vi "distance calculator.vi"(1 "Resolution Y":u16, 3 "Array":dbl[][](array[numeric])) -> (0 "Distances (Inches)":dbl)   [LabVIEW 2012]
doc: "Determines best target goal to calculate distance with, then uses bounding box top and bottom to calculate height. Determines distance by the formula:\ndistance = ( [ 1/2 ResolutionY * Goal size in inches] / Goal size in pixels ) / tan( 0.5 * Camera view angle)\nInputs: Goal Array (Portrait) & Image Resolution Y\nOutputs: Distance to Target (Inches)"
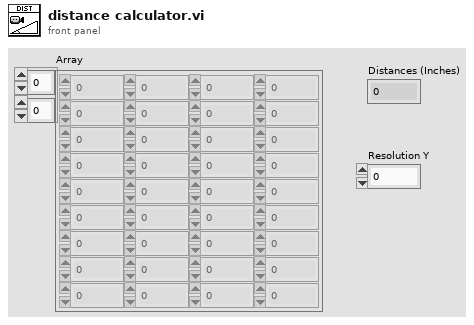
[diagram p1: front panel]
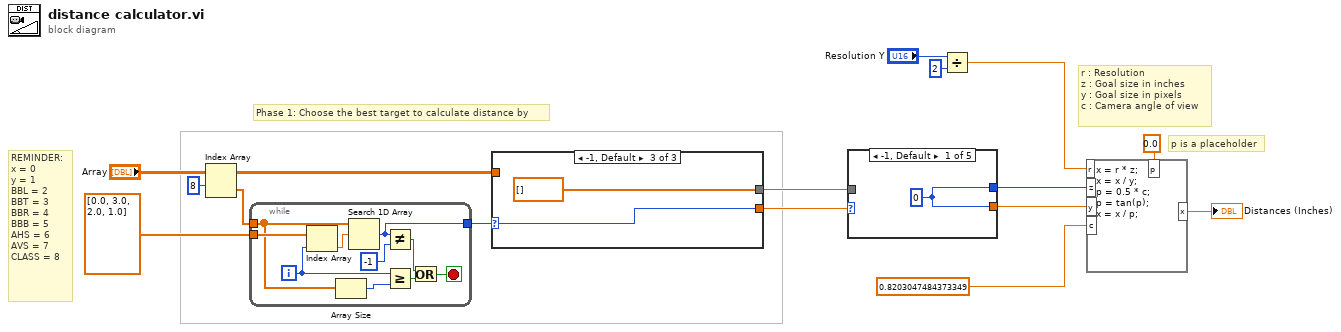
[diagram p0: block diagram]
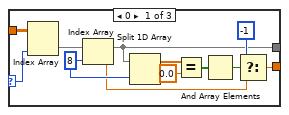
[diagram p2: hidden frame]
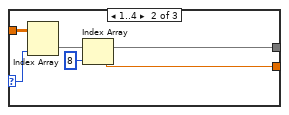
[diagram p3: hidden frame]
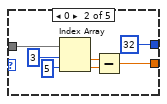
[diagram p4: hidden frame]
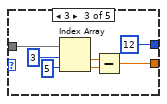
[diagram p5: hidden frame]
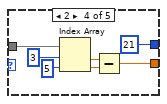
[diagram p6: hidden frame]
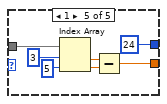
[diagram p7: hidden frame]
diagram:
  # "Phase 1: Choose the best target to calculate distance by"
  # "p is a placeholder"
  # "r : Resolution\nz : Goal size in inches\ny : Goal size in pixels\nc : Camera angle of view"
  # "REMINDER:\nx = 0\ny = 1\nBBL = 2\nBBT = 3\nBBR = 4 \nBBB = 5 \nAHS = 6\nAVS = 7 \nCLASS = 8"
  n1 = Index Array(array="Array", index (row)=8 ("disabled index (col)")) -> (element=w15:dbl[])  [unwired: 1 in]
  n2 = while {
    tunnel: w15 -> [w16]
    tunnel: dbl[] [0.0, 3.0, 2.0, 1.0] -> [w23]
    tunnel: [w24] -> w12
    i -> [w19]
    stop <- w21 stop-if-true
    n3 = Index Array(array=w23, index=w19) -> (element=w22:dbl)
    n4 = Array Size(array=w16) -> (size(s)=w18:i32)
    n5 = Search 1D Array(1D array=w16, element=w22) -> (index of element=w24:i32)  [unwired: 1 in]
    n6 = Not Equal?(x=w24, y=-1) -> (x != y?=w17:bool)
    n7 = Greater Or Equal?(x=w19, y=w18) -> (x >= y?=w20:bool)
    n8 = Or(x=w17, y=w20) -> (x .or. y?=w21:bool)
  }
  n9 = case shown="-1, Default" w12 {
    selector: w12 -> [w34 w39 w42]
    tunnel: "Array" -> [w35 w40 _]
    tunnel: [w28 w37 dbl[] [] ("Array")] -> w11
    tunnel: [w26 w38 w42] -> w5
    frame 0 {
      w33 = 8 ("index")
      n10 = Index Array(array=w35, index (col)=w34) -> (element=w28:dbl[])  [unwired: 1 in]
      n11 = Index Array(array=w28, index=w33) -> (element=w27:dbl)
      n12 = Split 1D Array(array=w28, index=w33) -> (first subarray=w32:dbl[])  [unwired: 1 out]
      n13 = Equal?(x=w32, y=0.0) -> (x = y?=w30:bool[])
      n14 = And Array Elements(Boolean array=w30) -> (logical AND=w29:bool)
      n15 = Select(t=-1, s=w29, f=w27) -> (s? t:f=w26:dbl)
    }
    frame 1..4 {
      n16 = Index Array(array=w40, index (col)=w39) -> (element=w37:dbl[])  [unwired: 1 in]
      n17 = Index Array(array=w37, index=8) -> (element=w38:dbl)
    }
    frame -1, Default {
    }
  }
  n18 = case shown="-1, Default" w5 {
    tunnel: w11 -> [_ w51 w58 w65 w72]
    tunnel: [w44 w46 w53 w60 w67] -> w10
    tunnel: [w44 32 12 21 24] -> w9
    frame -1, Default {
      w44 = 0
    }
    frame 0 {
      n19 = Index Array(array=w51, index #1=3, index #2=5) -> (element #1=w48:dbl, element #2=w47:dbl)
      n20 = Subtract(x=w48, y=w47) -> (x-y=w46:dbl)
    }
    frame 3 {
      n21 = Index Array(array=w58, index #1=3, index #2=5) -> (element #1=w55:dbl, element #2=w54:dbl)
      n22 = Subtract(x=w55, y=w54) -> (x-y=w53:dbl)
    }
    frame 2 {
      n23 = Index Array(array=w65, index #1=3, index #2=5) -> (element #1=w62:dbl, element #2=w61:dbl)
      n24 = Subtract(x=w62, y=w61) -> (x-y=w60:dbl)
    }
    frame 1 {
      n25 = Index Array(array=w72, index #1=3, index #2=5) -> (element #1=w69:dbl, element #2=w68:dbl)
      n26 = Subtract(x=w69, y=w68) -> (x-y=w67:dbl)
    }
  }
  n27 = Divide(x="Resolution Y", y=u16 2) -> (x/y=w3:dbl)
  n28 = formula code="x = r * z;\nx = x / y;\np = 0.5 * c;\np = tan(p);\nx = x / p;"("z"=w9, "r"=w3, "y"=w10, "c"=0.8203047484373349 ("input variable"), "p"=0.0 ("input variable")) -> ("x"=→"Distances (Inches)":dbl)
